vi "LED Immediate.vi"(7 "Description":string, 8 "Command Info In":T2, 9 "Color Box":u32(colorbox), 10 "Operation":T1, 11 "Sine Wave":dbl) -> (0 "Command Info Out":T2)   [LabVIEW 2025]
doc: "This template is useful for immediate subsystem actions that do not need deadband filtering\n\nBe sure to right-click and select New from Template and save with a new command name."
uses:
  <vilib>/Rock Robotics/WPI/Framework/Command Status Info.ctl
  <vilib>/Rock Robotics/WPI/Framework/Completion Status.ctl
  <vilib>/Rock Robotics/WPI/Framework/Completion Notifier.ctl
  Implementation/LEDs Operations.ctl
  Implementation/LEDs Setpoints.ctl
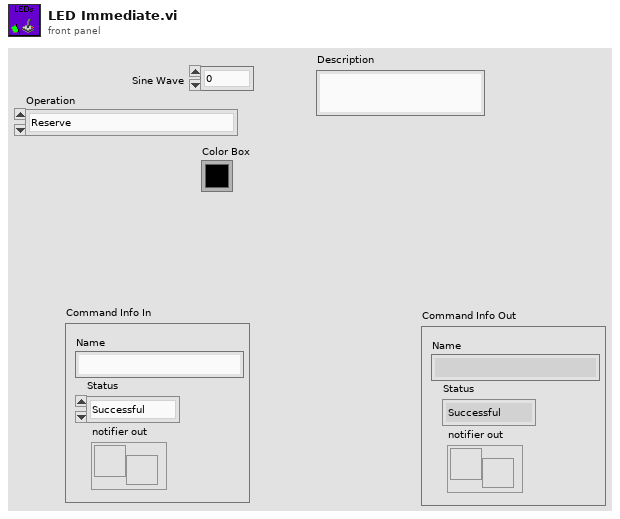
[diagram p1: front panel]
types:
  T1 = typedef "LEDs Operations.ctl" = enum16{"Reserve", "Read Current", "Immediate", "No Game Data", "Game Period", "Set Color"}
  T2 = typedef "Command Status Info.ctl" = cluster{"Name":string, "Status":T3, "notifier out":T4}
  T3 = typedef "Completion Status.ctl" = enum16{"Successful", "Aborted", "Incomplete"}
  T4 = typedef "Completion Notifier.ctl" = refnum<notifier>
  T5 = typedef "LEDs Setpoints.ctl" = cluster{"Operation":T1, "Sine Wave":dbl, "Time ":dbl, "Color Box":u32}
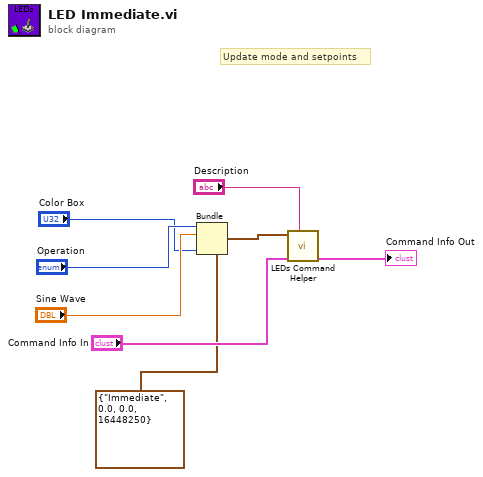
[diagram p0: block diagram]
diagram:
  # "Update mode and setpoints"
  n1 = Bundle(cluster=T5 {"Operation"=enum."Immediate", "Sine Wave"=0.0, "Time "=0.0, "Color Box"=16448250} ("SubSystem Data"), "Operation"="Operation", "Sine Wave"="Sine Wave", "Color Box"="Color Box") -> (w3:T5)  [unwired: 1 in]
  n2 = call "LEDs Command Helper.vi"("Description"="Description", "Command Info In"="Command Info In", "SubSystem Data"=w3) -> ("Command Info Out"=→"Command Info Out":T2)  [unwired: 6 in, 2 out]
